vi "Get All Scripts.vi"(7 "Server Alias":string, 10 "Error In":errorcluster) -> (2 "Error Out":errorcluster, 3 "All Scripts":T1[](array[typedef]))   [LabVIEW 2013, in "TS.lvlib"]
uses:
  TS.lvlib
  LabVIEW Example/Supporting Code/Script Running.ctl
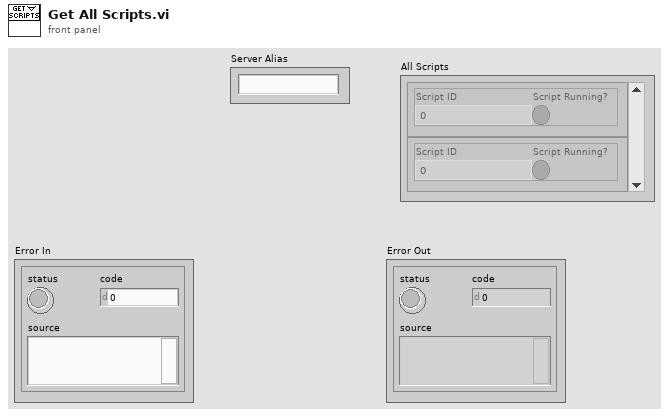
[diagram p1: front panel]
types:
  T1 = typedef "TS.lvlib/Script Running.ctl" = cluster{"Script ID":i64, "Script Running?":bool}
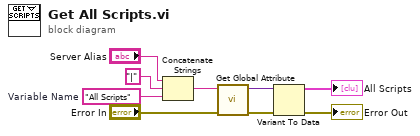
[diagram p0: block diagram]
diagram:
  w2 = "All Scripts"  # Variable Name
  n1 = Concatenate Strings("Server Alias", "|" ("string"), w2) -> (w1:string)
  n2 = call "Get Global Attribute.vi"("Error In"="Error In", "Name"=w1) -> ("Error Out"=w9:errorcluster, "Value"=w8:variant)  [unwired: 7 in, 1 out]
  n3 = Variant To Data(error in=w9, Variant=w8) -> (data=→"All Scripts":T1[], error out=→"Error Out":errorcluster)  [unwired: 1 in]
